vi "RT_Force mode_Oct19.vi"() -> ()   [LabVIEW 2018]
uses:
  <vilib>/Platform/TimedLoop/XDataNode/timing_clust.ctl
  <vilib>/Platform/TimedLoop/XDataNode/nitl_modes.ctl
  <vilib>/Platform/TimedLoop/XDataNode/wakeup.ctl
  <vilib>/FPGAPlugInAG/myRIO-1900/niLvFpga_Open_myRIO-1900.vi
  <vilib>/rvi/interface/common/dynamic/niFpgaDynamicAddResources.vi
  <vilib>/Utility/error.llb/Error Cluster From Error Code.vi
  <vilib>/rvi/errors/niLvFpgaAdjustHostInterfaceError.vi
  <vilib>/FPGAPlugInAG/Dynamic/niLvFpga_Close_Dynamic.vi
  <vilib>/rvi/interface/nirviOpenFPGA/nirviOpenFPGA.xnode
  UNCC Watt balance Oct19/FPGA Bitfiles/UNCCWattbalanceO_FPGATarget_fpgaW&RADCW2DACs_bUgWeZ5fmbw.lvbitx
  FPGA files/fpga_W&R_ADC_W_2DACs_Write_then_CLK.vi
  <vilib>/Platform/TimedLoop/XDataNode/XDataNode.xnode
  <vilib>/rvi/interface/nirviReadWriteControl/nirviReadWriteControl.xnode
  <vilib>/rvi/interface/nirviCloseFPGA/nirviCloseFPGA.xnode
  NiFpgaLv.dll
  <vilib>/rvi/interface/Simulation/niFpgaSimulationCallBeginRW.vi
  <vilib>/Platform/TimedLoop/XDataNode/XDNodeRunTimeDep.lvlib
panel:
  in  "PID":bool
  in  "Voltage to VC":dbl
  in  "Tare Value (gm)":dbl
  in  "TARE":bool
  in  "CH4":bool[](array[boolean])=[FALSE, FALSE, TRUE, TRUE, FALSE, TRUE, FALSE, FALSE, FALSE, FALSE, FALSE, FALSE, FALSE, FALSE, FALSE, FALSE]
  in  "gain":dbl=2.497 format="%#_13g"
  out "Current":dbl(graph)=0.004164202043930021
  out "mass":dbl(graph)=0.005695547840160359
  out "Finished Late? [i-1]":bool
  in  "delay (us)":i64=250
  out "Sample+Tare mass (gm)":dbl=0.005695547840160359 format="%.1g"
  in  "BL":dbl=13.4
  out "no. moving avg. Vsense":u8=50
  out "init array_moving avg. Vsense":dbl[](array[numeric])
  out "avg loop rate":dbl=3.8560259344012207
  out "error (nm)":dbl(graph)=-2.1361978729572595
  out "Voltage out":dbl(knob)=0.04046564536063808 scale=-10.0..10.0
  out "Displacement (um)":dbl(graph)=0.0021361978729572597
  in  "Stop Button":bool
  in  "setpoint (um)":dbl
  in  "KI":dbl=-0.0001 format="%#_13g"
  in  "Kp":dbl format="%#_13g"
  out "init array_moving avg. Z":dbl[](array[numeric])
  in  "no. moving avg. Z":u8=50
  in  "CH1":bool[](array[boolean])=[FALSE, FALSE, FALSE, FALSE, FALSE, TRUE, FALSE, FALSE, FALSE, FALSE, FALSE, FALSE, FALSE, FALSE, FALSE, FALSE]
  # "positive values move the stage towards table\nnegative valuesmove the stage away fromtable"
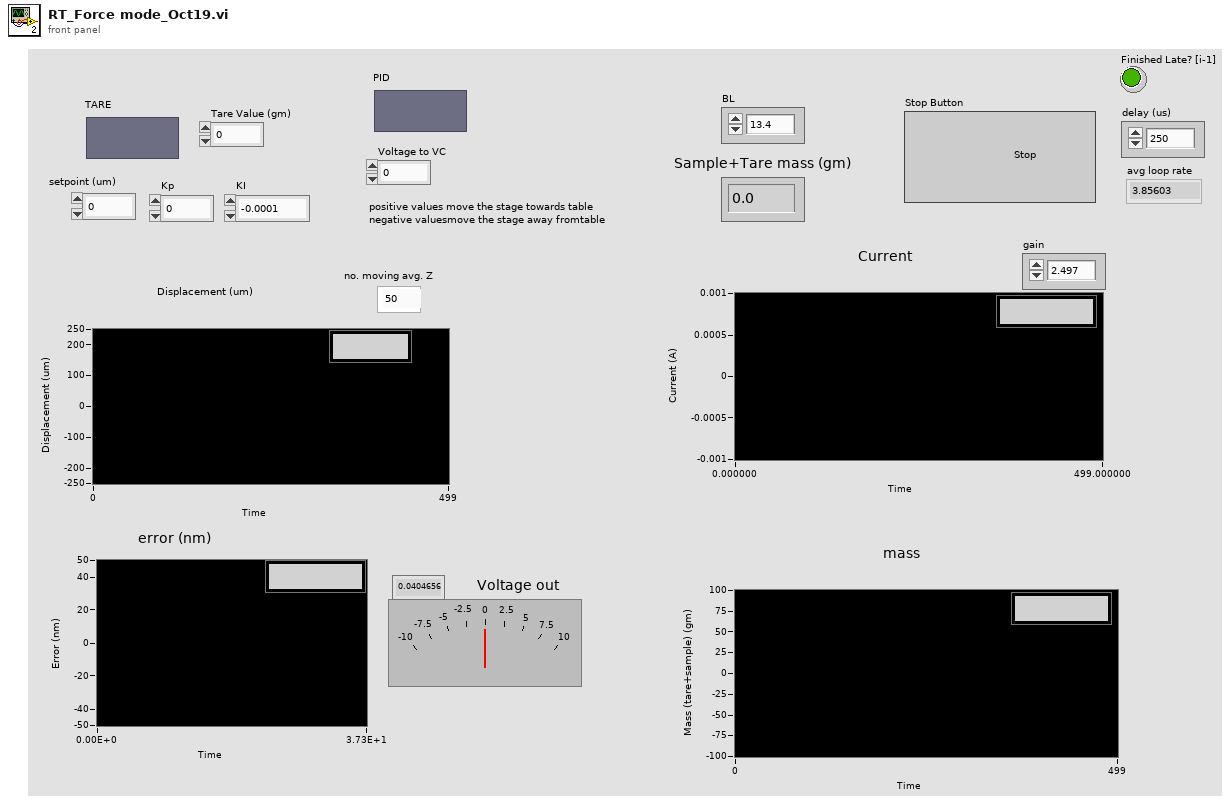
[diagram p1: front panel]
types:
  T1 = typedef "XDNodeRunTimeDep.lvlib/timing_clust.ctl" = cluster{"Expected End [f-1]":u64, "Actual End [f-1]":u64, "Finished Late? [f-1]":bool, "Expected End [i-1]":u64, "Actual End [i-1]":u64, "Finished Late? [i-1]":bool, "Expected Start [i]":u64, "Actual Start [i]":u64, "Expected Start [f]":u64, "Actual Start [f]":u64, "Source Name":string, "Structure Name":string, "Period":i64, "Deadline":i64, "Offset":i64, "Start":i64, "Priority":i32, "Timeout":i32, "Mode":T2, "Wakeup Reason":T3, "Error":errorcluster, "Source Type":string, "Secondary Source Type":string, "Global End Time":u64, "Global Start Time":u64, "Frame Duration":u64, "Iteration Duration":u64, "Assigned CPU":i32, "I/O Scan Engine Mode":u32}
  T2 = typedef "XDNodeRunTimeDep.lvlib/nitl_modes.ctl" = enum32{"No Change", "Process missed periods, maintain original phase", "Discard missed periods, maintain original phase", "Process missed periods, ignore original phase", "Discard missed periods, ignore original phase"}
  T3 = typedef "XDNodeRunTimeDep.lvlib/wakeup.ctl" = enum32{"Normal", "Aborted", "Asynchronous wakeup", "Timing source error", "Timed loop error", "Timeout"}
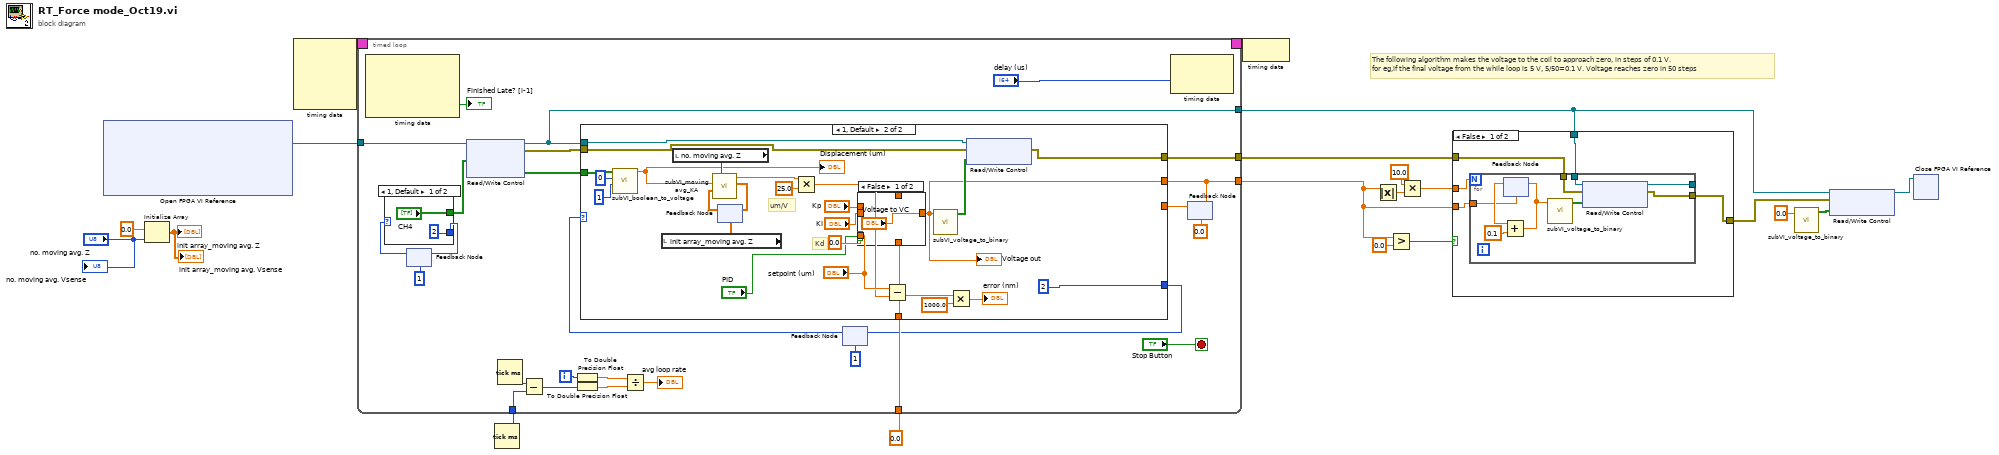
[diagram p0: block diagram]
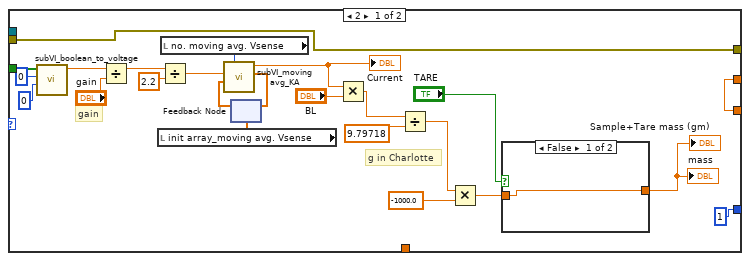
[diagram p2: hidden frame]
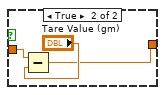
[diagram p3: hidden frame]
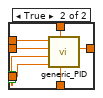
[diagram p4: hidden frame]
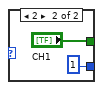
[diagram p5: hidden frame]
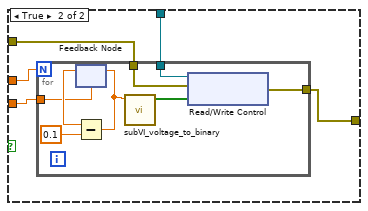
[diagram p6: hidden frame]
diagram:
  # "The following algorithm makes the voltage to the coil to approach zero, in steps of 0.1 V.\nfor eg,if the final voltage from the while loop is 5 V, 5/50=0.1 V. Voltage reaches zero in 50 steps"
  n1 = xnode "Open FPGA VI Reference"() -> ("FPGA VI Reference Out"=w7:refnum<k20>)  [unwired: 2 in, 1 out]
  n2 = Initialize Array(0.0 ("element"), "no. moving avg. Z") -> (→"init array_moving avg. Z" →"init array_moving avg. Vsense":dbl[])
  n3 = node-c288() -> (w20:T1)  [unwired: 4 in]
  n4 = Tick Count (ms)() -> (millisecond timer value=w8:u32)
  n5 = timed-loop {
    tunnel: w7 -> [w45]
    tunnel: [w30] -> w17
    tunnel: w8 -> [w39]
    tunnel: 0.0 ("initiation") -> [w37]
    timing: w20 -> [_]
    timing-out: [_] -> w19
    tunnel: [w25] -> w15
    tunnel: [w21] -> w5
    i -> [w38]
    stop <- "Stop Button" stop-if-true
    n6 = node-c288() -> (→"Finished Late? [i-1]":bool)  [unwired: 1 in, 3 out]
    n7 = feedback #1(1) -> (w36:i32)
    n8 = case shown="1, Default" w36 {
      tunnel: ["CH4" "CH1"] -> w22
      tunnel: [2 1] -> w34
      frame 1, Default {
      }
      frame 2 {
      }
    }
    n9 = feedback-in #1(w34) -> ()
    n10 = xnode "Read/Write Control"("FPGA VI Reference In"=w45, "ADC write"=w22) -> ("FPGA VI Reference Out"=w21:refnum<k20>, "error out"=w24:errorcluster, "ADC read"=w23:bool[])  [unwired: 1 in]
    n11 = Tick Count (ms)() -> (millisecond timer value=w40:u32)
    n12 = Subtract(x=w40, y=w39) -> (x-y=w44:u32)
    n13 = To Double Precision Float(number=w38) -> (double precision float=w42:dbl)
    n14 = To Double Precision Float(number=w44) -> (double precision float=w41:dbl)
    n15 = Divide(x=w42, y=w41) -> (x/y=→"avg loop rate":dbl)
    n16 = feedback #2(1) -> (w32:i32)
    n17 = node-c288("delay (us)") -> ()  [unwired: 1 in, 1 out]
    n18 = feedback #3(0.0 ("PID")) -> (w29:dbl)
    n19 = case shown="1, Default" w32 {
      tunnel: w21 -> [_ w82]
      tunnel: [w67 w95] -> w30
      tunnel: w37 -> [_ w92]
      tunnel: [1 2] -> w33
      tunnel: w29 -> [w67 _]
      tunnel: [w61 w87] -> w25
      tunnel: w24 -> [w61 w83]
      tunnel: w23 -> [w59 w84]
      frame 2 {
        # "gain"
        # "g in Charlotte"
        n20 = call "subVI_boolean_to_voltage.vi"("Gain"=i16 0, "UNI"=i16 0, "ADC read"=w59) -> ("V"=w60:dbl)  [unwired: 8 in]
        n21 = Divide(x=w60, y="gain") -> (x/y=w63:dbl)
        n22 = local read "init array_moving avg. Vsense"() -> (w72:dbl[])
        n23 = Divide(x=w63, y=2.2) -> (x/y=w69:dbl)
        n24 = local read "no. moving avg. Vsense"() -> (w74:u8)
        n25 = feedback #4(w72) -> (w73:dbl[])
        n26 = call "subVI_moving avg_KA.vi"("input array"=w73, "sample"=w69, "no. moving avg."=w74) -> ("output array"=w71:dbl[], "avg."=w62:dbl)  [unwired: 7 in]
        "Current" <- w62
        n27 = feedback-in #4(w71) -> ()
        n28 = Multiply(x=w62, y="BL") -> (x*y=w66:dbl)
        n29 = Divide(x=w66, y=9.79718) -> (x/y=w55:dbl)
        n30 = Multiply(x=w55, y=-1000.0) -> (x*y=w53:dbl)
        n31 = case shown="False" "TARE" {
          tunnel: w53 -> [w76 w79]
          tunnel: [w76 w77] -> w52
          frame False {
          }
          frame True {
            n32 = Subtract(x=w79, y="Tare Value (gm)") -> (x-y=w77:dbl)
          }
        }
        "Sample+Tare mass (gm)" <- w52
        "mass" <- w52
      }
      frame 1, Default {
        # "Kd"
        # "um/V"
        n33 = call "subVI_boolean_to_voltage.vi"("Gain"=i16 1, "UNI"=i16 0, "ADC read"=w84) -> ("V"=w80:dbl)  [unwired: 8 in]
        "Displacement (um)" <- w80
        n34 = local read "init array_moving avg. Z"() -> (w102:dbl[])
        n35 = local read "no. moving avg. Z"() -> (w103:u8)
        n36 = feedback #5(w102) -> (w104:dbl[])
        n37 = call "subVI_moving avg_KA.vi"("input array"=w104, "sample"=w80, "no. moving avg."=w103) -> ("output array"=w105:dbl[], "avg."=w100:dbl)  [unwired: 7 in]
        n38 = feedback-in #5(w105) -> ()
        n39 = Multiply(x=w100, y=25.0) -> (x*y=w93:dbl)
        n40 = case shown="False" "PID" {
          tunnel: "Kp" -> [_ w113]
          tunnel: "KI" -> [_ w112]
          tunnel: 0.0 ("Kd") -> [_ w111]
          tunnel: ["Voltage to VC" w110] -> w95
          tunnel: "setpoint (um)" -> [_ w109]
          tunnel: w93 -> [_ w108]
          tunnel: w92 -> [_ w107]
          frame False {
          }
          frame True {
            n41 = call "generic_PID.vi"("initiation"=w107, "sensor input"=w108, "setpoint"=w109, "Kd"=w111, "KI"=w112, "Kp"=w113) -> ("PID"=w110:dbl)  [unwired: 5 in]
          }
        }
        "Voltage out" <- w95
        n42 = Subtract(x="setpoint (um)", y=w93) -> (x-y=w90:dbl)
        n43 = call "subVI_voltage_to_binary.vi"("voltage"=w95) -> ("binary"=w96:bool[])  [unwired: 10 in]
        n44 = Multiply(x=w90, y=1000.0) -> (x*y=→"error (nm)":dbl)
        n45 = xnode "Read/Write Control"("FPGA VI Reference In"=w82, "error in"=w83, "DAC 2 write"=w96) -> ("error out"=w87:errorcluster)  [unwired: 1 out]
      }
    }
    n46 = feedback-in #2(w33) -> ()
    n47 = feedback-in #3(w30) -> ()
  }
  n48 = node-c288(w19) -> ()
  n49 = Absolute Value(x=w17) -> (abs(x)=w12:dbl)
  n50 = Greater?(x=w17, y=0.0) -> (0:w18:bool)
  n51 = Multiply(x=10.0, y=w12) -> (x*y=w16:dbl)
  n52 = case shown="False" w18 {
    tunnel: w16 -> [w122 w136]
    tunnel: w17 -> [w121 w135]
    tunnel: w15 -> [w120 w134]
    tunnel: w5 -> [w119 w133]
    tunnel: [w118 w132] -> w1
    frame False {
      n53 = for {
        N: w122 -> [_]
        tunnel: [w130] -> _
        tunnel: w121 -> [w127]
        tunnel: w120 -> [w125]
        tunnel: [w124] -> w118
        tunnel: w119 -> [w123]
        n54 = feedback #6(w127) -> (w128:dbl)
        n55 = Add(x=w128, y=0.1) -> (x+y=w126:dbl)
        n56 = feedback-in #6(w126) -> ()
        n57 = call "subVI_voltage_to_binary.vi"("voltage"=w126) -> ("binary"=w131:bool[])  [unwired: 10 in]
        n58 = xnode "Read/Write Control"("FPGA VI Reference In"=w123, "error in"=w125, "DAC 2 write"=w131) -> ("FPGA VI Reference Out"=w130:refnum<k20>, "error out"=w124:errorcluster)
      }
    }
    frame True {
      n59 = for {
        N: w136 -> [_]
        tunnel: w135 -> [w141]
        tunnel: w134 -> [w139]
        tunnel: [w138] -> w132
        tunnel: w133 -> [w137]
        n60 = feedback #7(w141) -> (w143:dbl)
        n61 = Subtract(x=w143, y=0.1) -> (x-y=w140:dbl)
        n62 = feedback-in #7(w140) -> ()
        n63 = call "subVI_voltage_to_binary.vi"("voltage"=w140) -> ("binary"=w144:bool[])  [unwired: 10 in]
        n64 = xnode "Read/Write Control"("FPGA VI Reference In"=w137, "error in"=w139, "DAC 2 write"=w144) -> ("error out"=w138:errorcluster)  [unwired: 1 out]
      }
    }
  }
  n65 = call "subVI_voltage_to_binary.vi"("voltage"=0.0) -> ("binary"=w3:bool[])  [unwired: 10 in]
  n66 = xnode "Read/Write Control"("FPGA VI Reference In"=w5, "error in"=w1, "DAC 2 write"=w3) -> ("FPGA VI Reference Out"=w4:refnum<k20>)  [unwired: 1 out]
  n67 = xnode "Close FPGA VI Reference"("FPGA VI Reference In"=w4) -> ()  [unwired: 1 in, 1 out]
  "no. moving avg. Vsense" <- "no. moving avg. Z"
